vi "h5_2D_I16.vi"(6 "Attributes":variant, 7 "TYPE":string="CAM", 8 "error in (no error)":errorcluster, 9 "2D I16":i16[][](array[numeric]), 10 "SQUID":string, 11 "H5":path[](array[path])) -> (0 "error out":errorcluster, 1 "Repeat":i32, 2 "Exists":bool)   [LabVIEW 2013]
uses:
  <vilib>/addons/h5labview2/file/H5Fmode.ctl
  <vilib>/addons/h5labview2/base/lib_path.vi
  <vilib>/addons/h5labview2/base/H5Equery.vi
  <vilib>/addons/h5labview2/base/hid_t.ctl
  <vilib>/addons/h5labview2/dataset/H5Dwrite.llb/H5Dwrite.xnode
  <vilib>/addons/h5labview2/file/H5F.lvlib
  <vilib>/addons/h5labview2/group/H5G.lvlib
  <vilib>/addons/h5labview2/attrib/H5A.lvlib
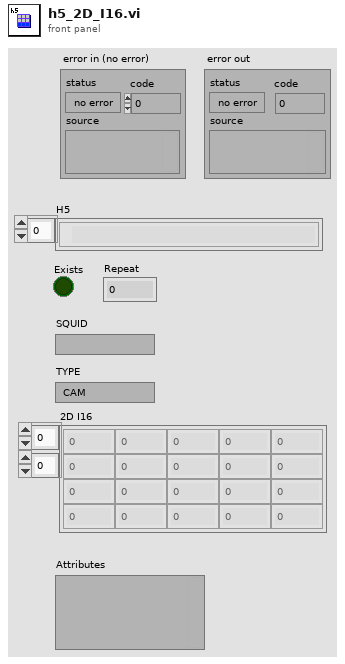
[diagram p1: front panel]
types:
  T1 = typedef "Semaphore RefNum" = refnum<k1>
  T2 = typedef "H5F.lvlib/H5Fmode.ctl" = enum16{"read-only", "read-write", "overwrite", "create new", "open or create"}
  T3 = typedef "hid_t.ctl" = i32
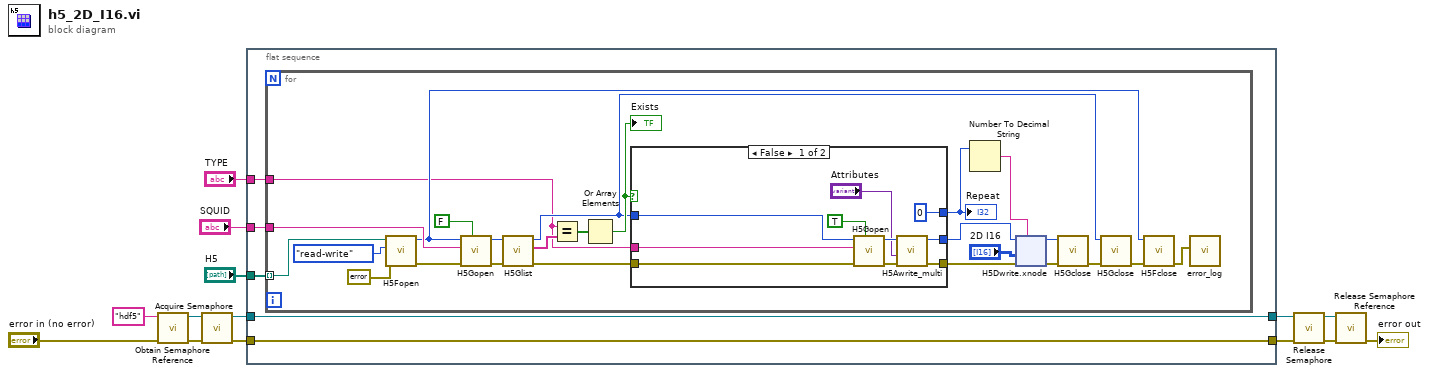
[diagram p0: block diagram]
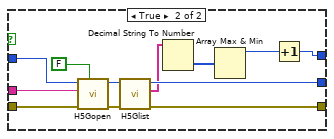
[diagram p2: hidden frame]
diagram:
  n1 = call <vilib>:"Obtain Semaphore Reference.vi"("error in (no error)"="error in (no error)", "name (unnamed)"="hdf5") -> ("error out"=w13:errorcluster, "semaphore"=w14:T1)  [unwired: 3 in, 1 out]
  n2 = call <vilib>:"Acquire Semaphore.vi"("error in (no error)"=w13, "semaphore"=w14) -> ("error out"=w7:errorcluster, "semaphore out"=w6:T1)  [unwired: 3 in, 1 out]
  n3 = flat-sequence {
    tunnel: [w19] -> w8
    tunnel: w7 -> [w19]
    tunnel: w6 -> [w18]
    tunnel: [w18] -> w5
    tunnel: "H5" -> [w17]
    tunnel: "SQUID" -> [w16]
    tunnel: "TYPE" -> [w15]
    frame #0 {
      n4 = for {
        tunnel: w17 -> [w40] mode=indexing
        tunnel: w16 -> [w41]
        tunnel: w15 -> [w31]
        n5 = call <vilib>:"H5Fopen.vi"("error in (no error)"=errorcluster {"status"=FALSE, "code"=0, "source"=""}, "mode (read-only)"=H5Fmode."read-write", "path"=w40) -> ("error out"=w39:errorcluster, "ref out"=w38:T3)  [unwired: 7 in]
        n6 = call <vilib>:"H5Gopen.vi"("create? (F)"=FALSE, "error in (no error)"=w39, "name"=w41, "ref in"=w38) -> ("error out"=w36:errorcluster, "group out"=w37:T3)  [unwired: 6 in]
        n7 = call <vilib>:"H5Glist.vi"("error in (no error)"=w36, "ref in"=w37) -> ("error out"=w30:errorcluster, "names"=w35:string[], "ref out"=w32:T3)  [unwired: 6 in, 1 out]
        n8 = Equal?(x=w31, y=w35) -> (x = y?=w34:bool[])
        n9 = Or Array Elements(Boolean array=w34) -> (logical OR=w33:bool)
        "Exists" <- w33
        n10 = case shown="False" w33 {
          tunnel: w32 -> [w53 w63]
          tunnel: w31 -> [w52 w64]
          tunnel: w30 -> [w51 w65]
          tunnel: [w48 w61] -> w27
          tunnel: [w47 w59] -> w28
          tunnel: [0 w55] -> w22
          frame False {
            n11 = call <vilib>:"H5Gopen.vi"("create? (F)"=TRUE, "error in (no error)"=w51, "name"=w52, "ref in"=w53) -> ("error out"=w49:errorcluster, "group out"=w46:T3)  [unwired: 6 in]
            n12 = call <vilib>:"H5Awrite_multi.vi"("error in (no error)"=w49, "variant in"="Attributes", "ref in"=w46) -> ("error out"=w48:errorcluster, "ref out"=w47:T3)  [unwired: 7 in]
          }
          frame True {
            n13 = call <vilib>:"H5Gopen.vi"("create? (F)"=FALSE, "error in (no error)"=w65, "name"=w64, "ref in"=w63) -> ("error out"=w62:errorcluster, "group out"=w60:T3)  [unwired: 6 in]
            n14 = call <vilib>:"H5Glist.vi"("error in (no error)"=w62, "ref in"=w60) -> ("error out"=w61:errorcluster, "names"=w58:string[], "ref out"=w59:T3)  [unwired: 6 in, 1 out]
            n15 = Decimal String To Number(string=w58) -> (number=w57:i32[])  [unwired: 2 in, 1 out]
            n16 = Array Max & Min(array=w57) -> (max value=w56:i32)  [unwired: 3 out]
            n17 = Increment(x=w56) -> (x+1=w55:i32)
          }
        }
        "Repeat" <- w22
        n18 = Number To Decimal String(number=w22) -> (decimal integer string=w23:string)  [unwired: 1 in]
        n19 = xnode "H5Dwrite.xnode"("dataset name"=w23, "error in (no error)"=w27, "data"="2D I16", "ref in"=w28) -> ("error out"=w25:errorcluster, "ref out"=w26:T3)  [unwired: 3 in, 1 out]
        n20 = call <vilib>:"H5Gclose.vi"("error in (no error)"=w25, "group in"=w26) -> ("error out"=w24:errorcluster)  [unwired: 9 in]
        n21 = call <vilib>:"H5Gclose.vi"("error in (no error)"=w24, "group in"=w32) -> ("error out"=w42:errorcluster)  [unwired: 9 in]
        n22 = call <vilib>:"H5Fclose.vi"("error in (no error)"=w42, "ref"=w38) -> ("error out"=w21:errorcluster)  [unwired: 9 in]
        n23 = call "error_log.vi"("error"=w21) -> ()  [unwired: 10 in]
      }
    }
  }
  n24 = call <vilib>:"Release Semaphore.vi"("error in (no error)"=w8, "semaphore"=w5) -> ("error out"=w9:errorcluster, "semaphore out"=w10:T1)  [unwired: 4 in]
  n25 = call <vilib>:"Release Semaphore Reference.vi"("error in (no error)"=w9, "semaphore"=w10) -> ("error out"=→"error out":errorcluster)  [unwired: 8 in, 1 out]
